vi "Convert Lin Mag to dB.vi"(7 "convert to dB":bool, 8 "dB reference (ch Y)":dbl=1.0, 9 "dB reference (ch X)":dbl=1.0, 10 "spectrum type":T1(ring), 11 "magnitude H(w)":cluster{"f0":dbl, "df":dbl, "Mag H(w)":dbl[]}) -> (3 "magnitude H(w) in dB":cluster{"f0":dbl, "df":dbl, "Mag H(w)":dbl[]})   [LabVIEW 2023]
doc: "Convert Magnitude to dB."
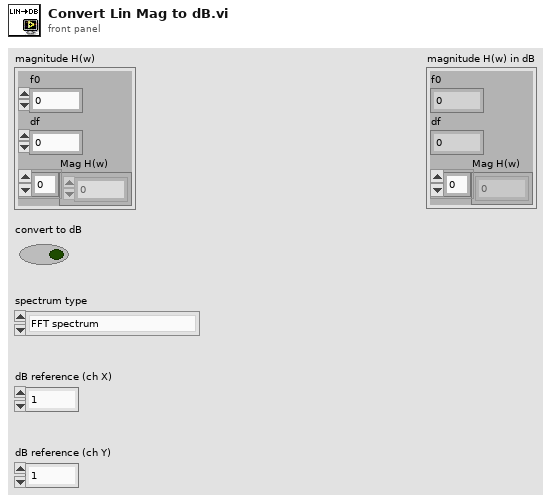
[diagram p1: front panel]
types:
  T1 = enum16{"FFT spectrum", "Power spectrum", "Cross spectrum", "Frequency response"}
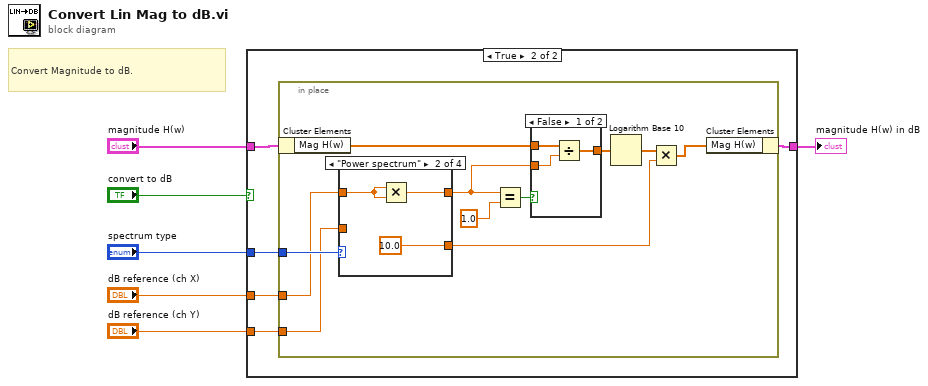
[diagram p0: block diagram]
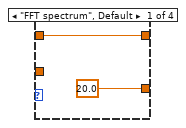
[diagram p4: hidden frame]
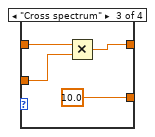
[diagram p5: hidden frame]
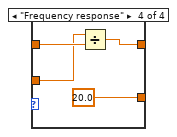
[diagram p6: hidden frame]
diagram:
  # "Convert Magnitude to dB."
  n1 = case shown="True" "convert to dB" {
    tunnel: "magnitude H(w)" -> [w7 w9]
    tunnel: [w7 w8] -> w5
    tunnel: "spectrum type" -> [_ w12]
    tunnel: "dB reference (ch X)" -> [_ w11]
    tunnel: "dB reference (ch Y)" -> [_ w10]
    frame False {
    }
    frame True {
      n2 = in-place {
        in-place-border: w12 -> [w23]
        in-place-border: w11 -> [w22]
        in-place-border: w10 -> [w21]
        n3 = in-place-cluster #1(w9) -> ("Mag H(w)"=w17:dbl[])
        n4 = case shown="\"Power spectrum\"" w23 {
          tunnel: w22 -> [w29 w31 w36 w40]
          tunnel: [w29 w32 w34 w39] -> w16
          tunnel: [20.0 10.0 10.0 20.0] -> w15
          tunnel: w21 -> [_ _ w35 w38]
          frame "FFT spectrum", Default {
          }
          frame "Power spectrum" {
            n5 = Multiply(x=w31, y=w31) -> (x*y=w32:dbl)
          }
          frame "Cross spectrum" {
            n6 = Multiply(x=w36, y=w35) -> (x*y=w34:dbl)
          }
          frame "Frequency response" {
            n7 = Divide(x=w38, y=w40) -> (x/y=w39:dbl)
          }
        }
        n8 = Equal?(x=w16, y=1.0) -> (x = y?=w18:bool)
        n9 = case shown="False" w18 {
          tunnel: w17 -> [w26 w27]
          tunnel: [w25 w27] -> w20
          tunnel: w16 -> [w24 _]
          frame False {
            n10 = Divide(x=w26, y=w24) -> (x/y=w25:dbl[])
          }
          frame True {
          }
        }
        n11 = Logarithm Base 10(1:w20) -> (0:w19:dbl[])
        n12 = Multiply(x=w19, y=w15) -> (x*y=w14:dbl[])
        n13 = in-place-cluster #1("Mag H(w)"=w14) -> (w8:cluster{"f0":dbl, "df":dbl, "Mag H(w)":dbl[]})
      }
    }
  }
  "magnitude H(w) in dB" <- w5
